vi "Store Last Config.vi"(8 "error in (no error)":errorcluster, 11 "Refnum in":T1) -> (0 "error out":errorcluster, 3 "Refnum out":T1)   [LabVIEW 2017]
uses:
  <vilib>/Utility/config.llb/Config Data RefNum.ctl
  <vilib>/Utility/config.llb/Read Key (String).vi
  <vilib>/Utility/config.llb/Write Key (String).vi
  <vilib>/Utility/config.llb/NI_LVConfig.lvlib
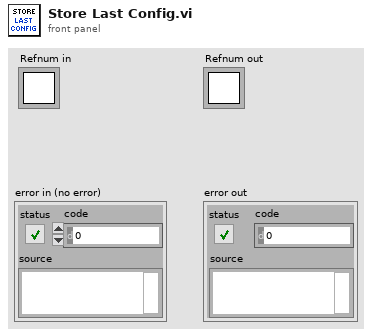
[diagram p1: front panel]
types:
  T1 = typedef "NI_LVConfig.lvlib/Config Data RefNum.ctl" = refnum<k1>
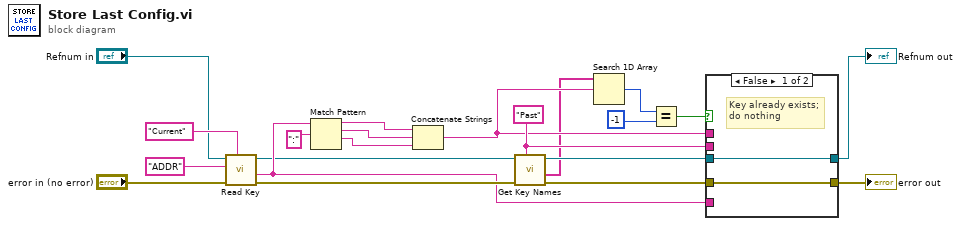
[diagram p0: block diagram]
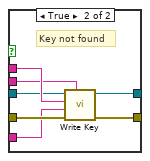
[diagram p2: hidden frame]
diagram:
  w7 = "Past"
  n1 = call-poly <vilib>:"Read Key.vi"("section"="Current", "error in (no error)"="error in (no error)", "key"="ADDR", "refnum"="Refnum in") -> ("error out"=w12:errorcluster, "value"=w10:string, "refnum out"=w9:T1)  [unwired: 4 in, 1 out]
  n2 = Match Pattern(string=w10, regular expression=":") -> (before substring=w1:string, match substring=w13:string, after substring=w14:string)  [unwired: 1 in, 1 out]
  n3 = Concatenate Strings(w1, w13, w14) -> (w6:string)
  n4 = call <vilib>:"Get Key Names.vi"("section"=w7, "error in (no error)"=w12, "refnum"=w9) -> ("error out"=w11:errorcluster, "key names"=w5:string[], "refnum out"=w8:T1)  [unwired: 5 in, 1 out]
  n5 = Search 1D Array(1D array=w5, element=w6) -> (index of element=w4:i32)  [unwired: 1 in]
  n6 = Equal?(x=w4, y=-1) -> (x = y?=w3:bool)
  n7 = case shown="False" w3 {
    tunnel: [w23 w30] -> w20
    tunnel: [w22 w29] -> w19
    tunnel: w6 -> [_ w28]
    tunnel: w11 -> [w23 w27]
    tunnel: w10 -> [_ w26]
    tunnel: w8 -> [w22 w25]
    tunnel: w7 -> [_ w24]
    frame False {
      # "Key already exists;\ndo nothing"
    }
    frame True {
      # "Key not found"
      n8 = call-poly <vilib>:"Write Key.vi"("section"=w24, "error in (no error)"=w27, "value"=w26, "key"=w28, "refnum"=w25) -> ("error out"=w30:errorcluster, "refnum out"=w29:T1)  [unwired: 4 in, 1 out]
    }
  }
  "Refnum out" <- w19
  "error out" <- w20
